vi "controller.vi"(3 "KD":sgl, 6 "Reset":bool, 7 "Parameters":T1={"Stimulus"={"Type"=enum."Off", "Phase"=0.0, "Amplitude"=[0.0, 0.0, 0.0], "Injection point"=enum."Total pose", "Closed loop"=FALSE, "Offset"=[0.0, 0.0, 0.0], "Tip -> world"=TRUE, "Frequency"=0.0, "Length"=0.0}, "Goal Filter A"={"Speedup max"=0.0, "Speedup thresh"=0.15, "Speedup nonlin"=0.0, "Filters"=[]}, "Mode controls"={"Hold"=FALSE, "Cancellation"=FALSE, "Goal filter"=FALSE, "Trigger"=FALSE}, "Manipulator type"=enum."Current piezo", "Manipulator calibration"={"Tool offsets"=[[-0.47364116, -0.25724307, -1.1087934], [0.29673597, -0.25864395, -1.0971603], [-0.04366469, 0.4463568, -1.1035515]], "Tip light calibration"=[[3.2813332, 0.23462732, 0.17832138, -8265.082], [-0.20249099, 2.693321, -0.28150028, -33565.66], [-0.1458117, 0.68216485, 0.8833545, 26862.188], [-1.1202011e-18, 5.861468e-19, 1.7601345e-18, 1.0]], "Handle light calibration"=[], "Base pivots"=[], "Output pivots"=[[0.0, 0.0, -11360.0]], "Length center"=0.0, "Workspace height"=[], "Workspace diameter"=[0.0, 0.0, 36200.0], "Linearization"=[], "Stack travel"=400.0, "Saturation pos"=375.0, "Inverse filters"=[]}, "Network"={"Remote Host"="", "Send Status"=FALSE, "Send Port"=50, "Recv Commands"=FALSE, "Recv Port"=0}, "Goal Filter B"={"Speedup max"=0.0, "Speedup thresh"=0.0, "Speedup nonlin"=0.0, "Filters"=[]}, "Cancellation"={"KP"={"XY"=0.0, "Rxy"=0.0, "Z"=0.0, "Rz"=0.0}, "KI"=2.0, "KD"={"XY"=0.0, "Rxy"=0.0, "Z"=0.0, "Rz"=0.0}, "Max vel"=20.0, "Max acc"=61557.0, "Int error limit"=2.0, "RCM gain"=0.0, "Bypass"=FALSE, "Degraded gain"=0.0}, "Transition time"=0.0, "Estimation"={"Link"={"Measure noise"=[], "Process noise"=[], "Alt process noise"=[], "Alt turnoff cycles"=20, "Innovation limit"=[], "Residue threshold"=0.0, "Enable"=FALSE}, "Handle"={"Measure noise"=[], "Process noise"=[], "State limits"=[], "Innovation limit"=[], "Prediction Lookahead"=0.0, "Enable"=FALSE}}} {"Transition time" format="%_3f"; "Cancellation"."Degraded gain" min=0 max=1 step=0.1 format="%#_3p"; "Cancellation"."RCM gain" min=0 max=1 step=0.1 format="%#_3p"; "Cancellation"."KD"."Rz" min=0 max=1 step=0.1 format="%#_3p"; "Cancellation"."KD"."Rxy" min=0 max=1 step=0.1 format="%#_3p"; "Cancellation"."KD"."Z" min=0 max=1 step=0.1 format="%#_3p"; "Cancellation"."KD"."XY" min=0 max=1 step=0.1 format="%#_3p"; "Cancellation"."KI" min=0 max=1 step=0.01 format="%#_3p"; "Cancellation"."KP"."Rz" min=0 max=1 step=0.1 format="%#_3p"; "Cancellation"."KP"."Rxy" min=0 max=1 step=0.1 format="%#_3p"; "Cancellation"."KP"."Z" min=0 max=1 step=0.1 format="%#_3p"; "Cancellation"."KP"."XY" min=0 max=1 step=0.1 format="%#_3p"; "Cancellation"."Max acc" format="%#_3p"; "Goal Filter B"."Filters"."V limit range" format="%_3p"; "Goal Filter B"."Filters"."V limit" format="%_3p"; "Goal Filter B"."Filters"."Upper Q" format="%_3f"; "Goal Filter B"."Filters"."Upper Fc" format="%_3p"; "Goal Filter B"."Filters"."Lower Q" format="%_3f"; "Goal Filter B"."Filters"."Scale factor" format="%_3f"; "Goal Filter B"."Filters"."Lower Fc" format="%_3p"; "Goal Filter B"."Speedup nonlin" format="%_3p"; "Goal Filter B"."Speedup thresh" format="%_3p"; "Goal Filter B"."Speedup max" format="%_3p"; "Manipulator calibration"."Saturation pos" format="%#.1f"; "Manipulator calibration"."Stack travel" format="%#.1f"; "Manipulator calibration"."Output pivots" format="%#_6f"; "Manipulator calibration"."Base pivots" format="%#_6f"; "Manipulator calibration"."Handle light calibration" format="%#.1f"; "Manipulator calibration"."Tip light calibration" format="%#.1f"; "Goal Filter A"."Filters"."V limit range" format="%_3p"; "Goal Filter A"."Filters"."V limit" format="%_3p"; "Goal Filter A"."Filters"."Upper Q" format="%_3f"; "Goal Filter A"."Filters"."Upper Fc" format="%_3p"; "Goal Filter A"."Filters"."Lower Q" format="%_3f"; "Goal Filter A"."Filters"."Scale factor" format="%_3f"; "Goal Filter A"."Filters"."Lower Fc" format="%_3p"; "Goal Filter A"."Speedup nonlin" format="%_3p"; "Goal Filter A"."Speedup thresh" format="%_3p"; "Goal Filter A"."Speedup max" format="%_3p"; "Stimulus"."Length" min=0.0 max=100.0 step=100.0 format="%#_4p"; "Stimulus"."Frequency" min=0.0 step=100.0 format="%#_4g"; "Stimulus"."Offset" format="%#_3p"; "Stimulus"."Amplitude" format="%#_3p"; "Stimulus"."Phase" min=-180.0 max=360.0 step=100.0 format="%#.2f"}, 8 "Manipulator status":sgl[](array[numeric]), 9 "KI":sgl, 10 "Stack error in":sgl[](array[numeric]), 11 "KP":sgl) -> (4 "Saturation":bool, 5 "Stack commands":sgl[](array[numeric]))   [LabVIEW 2013]
uses:
  testing/Micron params.ctl
  testing/stimulus.ctl
  testing/injection_point.ctl
  filtering/goal_loop_parms.ctl
  testing/mode_conrols.ctl
  testing/manipulator_cal.ctl
  asap/labview/testing/probe_calibration.ctl
  host/network_params.ctl
  sq_control_params.ctl
  decoupled_gain.ctl
  estimation_controls.ctl
panel:
  in  "Last stack error":sgl[](array[numeric])
  in  "Integral error":sgl[](array[numeric])=[0.0, 0.0, 0.0, 0.0, 0.0, 0.0]
  # "Locals:"
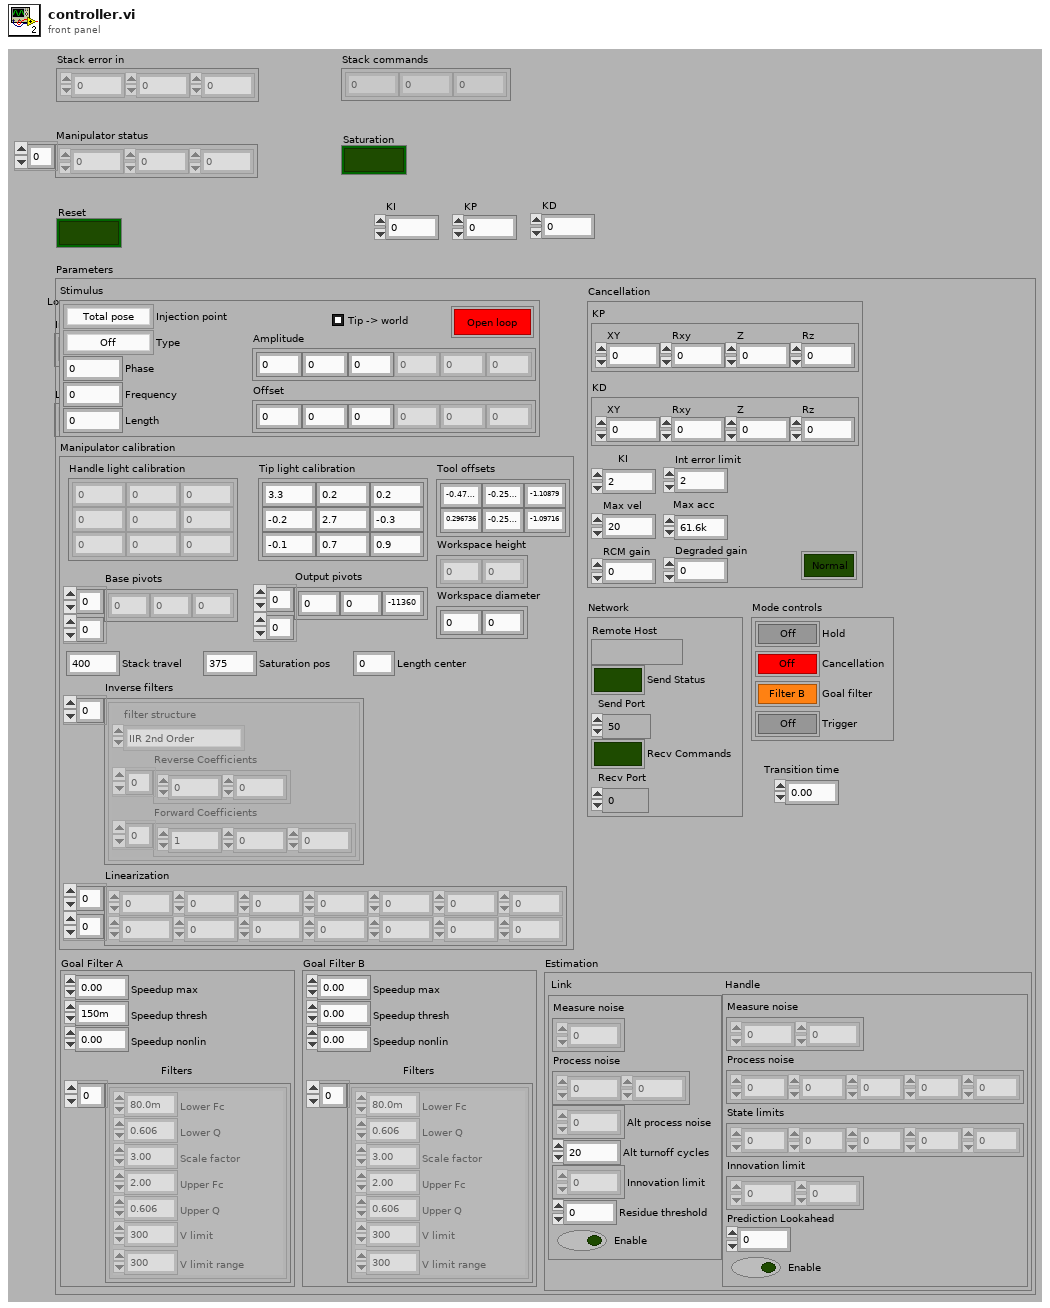
[diagram p1: front panel]
types:
  T1 = typedef "Micron params.ctl" = cluster{"Stimulus":T2, "Goal Filter A":T4, "Mode controls":T5, "Manipulator type":enum16{"Current piezo", "Voltage piezo"}, "Manipulator calibration":T6, "Network":T8, "Goal Filter B":T4, "Cancellation":T9, "Transition time":sgl, "Estimation":T11}
  T2 = typedef "stimulus.ctl" = cluster{"Type":enum16{"Off", "Step", "Sine", "Triangle", "Arbitrary"}, "Phase":dbl, "Amplitude":sgl[], "Injection point":T3, "Closed loop":bool, "Offset":sgl[], "Tip -> world":bool, "Frequency":dbl, "Length":dbl}
  T3 = typedef "injection_point.ctl" = enum16{"Total pose", "V limiter", "Goal ", "Link position", "KF link position", "Inverse kin", "Link goal", "Link error", "Controller", "Output", "Drive", "Light"}
  T4 = typedef "goal_loop_parms.ctl" = cluster{"Speedup max":sgl, "Speedup thresh":sgl, "Speedup nonlin":sgl, "Filters":cluster{"Lower Fc":sgl, "Lower Q":sgl, "Scale factor":sgl, "Upper Fc":sgl, "Upper Q":sgl, "V limit":sgl, "V limit range":sgl}[]}
  T5 = typedef "mode_conrols.ctl" = cluster{"Hold":bool, "Cancellation":bool, "Goal filter":bool, "Trigger":bool}
  T6 = typedef "manipulator_cal.ctl" = cluster{"Tool offsets":sgl[][], "Tip light calibration":T7, "Handle light calibration":T7, "Base pivots":sgl[][], "Output pivots":sgl[][], "Length center":sgl, "Workspace height":sgl[], "Workspace diameter":sgl[], "Linearization":sgl[][], "Stack travel":sgl, "Saturation pos":sgl, "Inverse filters":cluster{"filter structure":enum32{"IIR 2nd Order", "IIR 4th Order"}, "Reverse Coefficients":dbl[], "Forward Coefficients":dbl[]}[]}
  T7 = typedef "probe_calibration.ctl" = sgl[][]
  T8 = typedef "network_params.ctl" = cluster{"Remote Host":string, "Send Status":bool, "Send Port":u16, "Recv Commands":bool, "Recv Port":u16}
  T9 = typedef "sq_control_params.ctl" = cluster{"KP":T10, "KI":sgl, "KD":T10, "Max vel":sgl, "Max acc":sgl, "Int error limit":sgl, "RCM gain":sgl, "Bypass":bool, "Degraded gain":sgl}
  T10 = typedef "decoupled_gain.ctl" = cluster{"XY":sgl, "Rxy":sgl, "Z":sgl, "Rz":sgl}
  T11 = typedef "estimation_controls.ctl" = cluster{"Link":cluster{"Measure noise":dbl[], "Process noise":dbl[], "Alt process noise":dbl[], "Alt turnoff cycles":i32, "Innovation limit":dbl[], "Residue threshold":dbl, "Enable":bool}, "Handle":cluster{"Measure noise":dbl[], "Process noise":dbl[], "State limits":dbl[], "Innovation limit":dbl[], "Prediction Lookahead":sgl, "Enable":bool}}
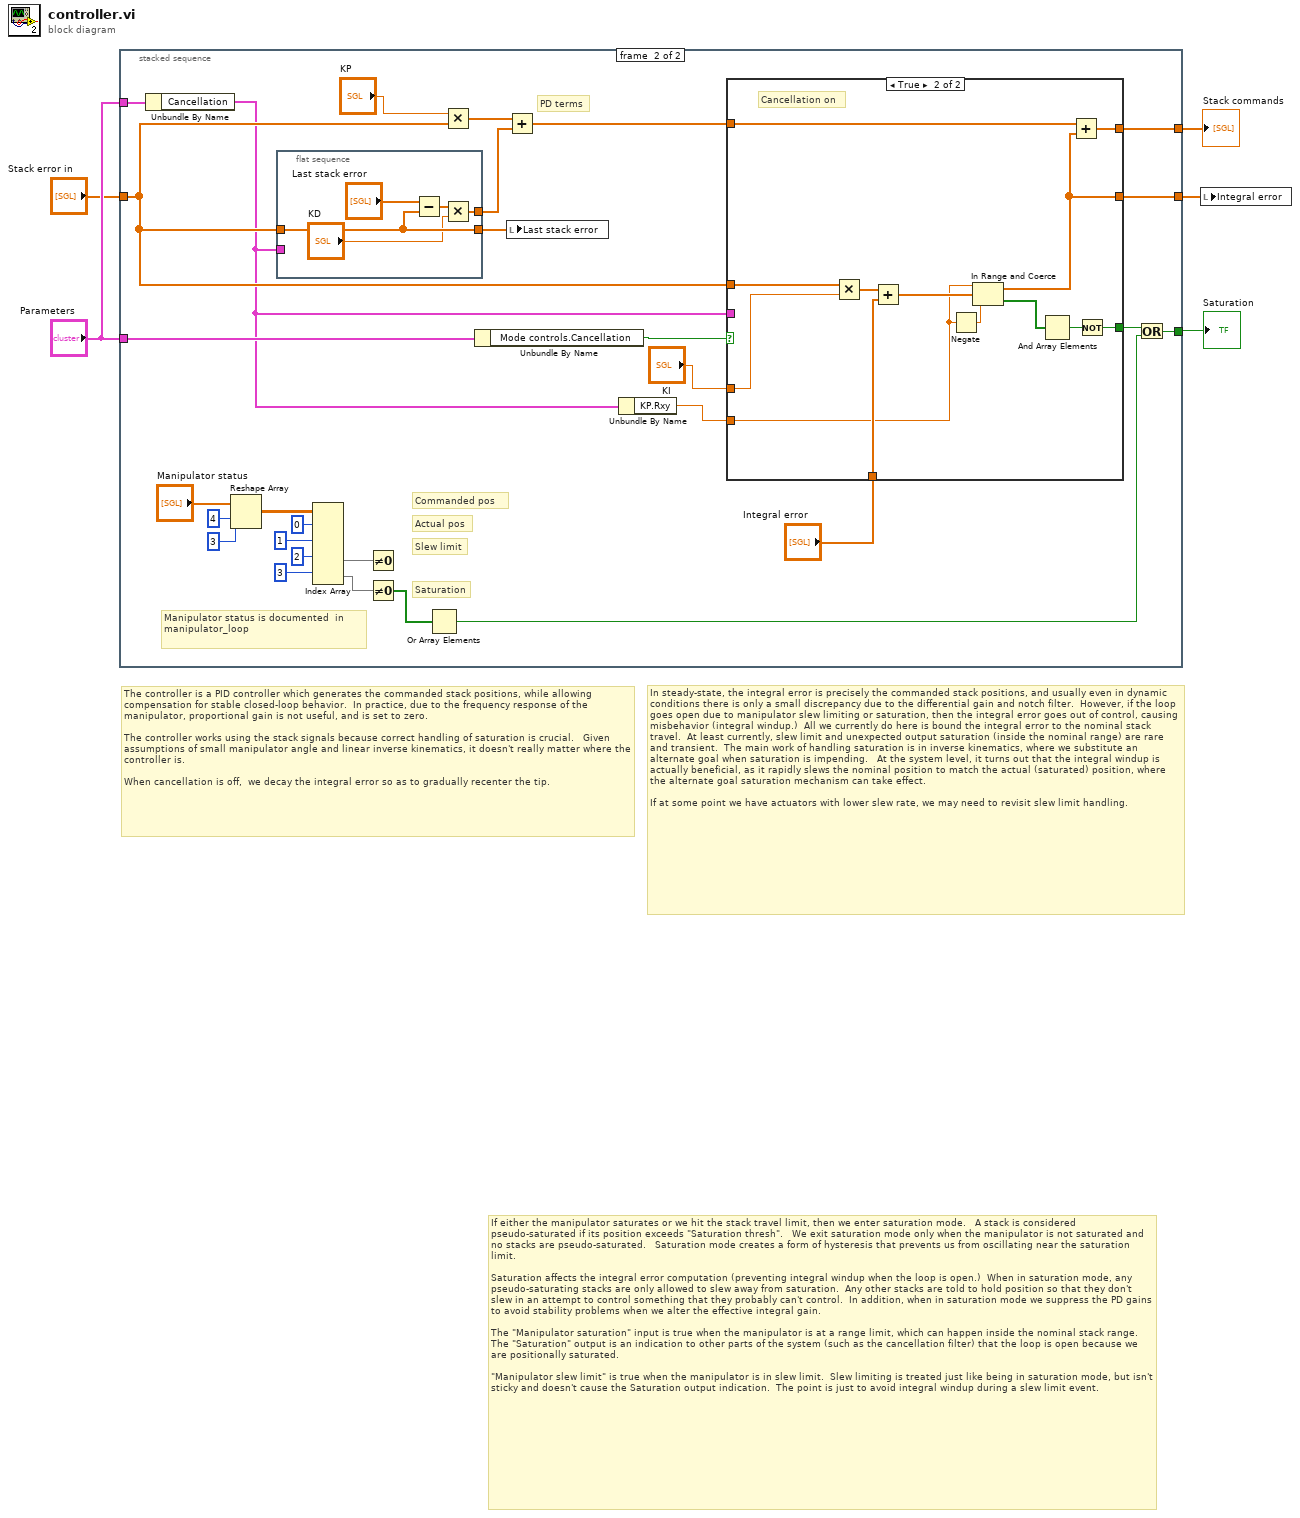
[diagram p0: block diagram]
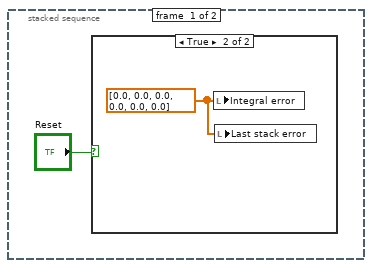
[diagram p2: hidden frame]
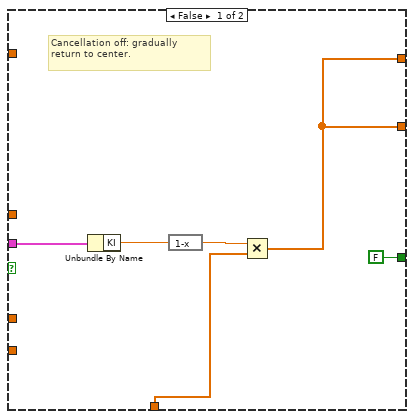
[diagram p4: hidden frame]
diagram:
  # "In steady-state, the integral error is precisely the commanded stack positions, and usually even in dynamic conditions there is only a small discrepancy due to the differential gain and notch filter.  However, if the loop goes open due to manipulator slew limiting or saturation, then the integral error goes out of control, causing  misbehavior (integral windup.)  All we currently do here is bound the integral error to the nominal stack travel.  At least currently, slew limit and unexpected output saturation (inside the nominal range) are rare and transient.  The main work of handling saturation is in inverse kinematics, where we substitute an alternate goal when saturation is impending.   At the system level, it turns out that the integral windup is actually beneficial, as it rapidly slews the nominal position to match the actual (saturated) position, where the alternate goal saturation mechanism can take effect.\n\nIf at some point we have actuators with lower slew rate, we may need to revisit slew limit handling."
  # "If either the manipulator saturates or we hit the stack travel limit, then we enter saturation mode.   A stack is considered pseudo-saturated if its position exceeds \"Saturation thresh\".   We exit saturation mode only when the manipulator is not saturated and no stacks are pseudo-saturated.   Saturation mode creates a form of hysteresis that prevents us from oscillating near the saturation limit.  \n\nSaturation affects the integral error computation (preventing integral windup when the loop is open.)  When in saturation mode, any  pseudo-saturating stacks are only allowed to slew away from saturation.  Any other stacks are told to hold position so that they don't slew in an attempt to control something that they probably can't control.  In addition, when in saturation mode we suppress the PD gains to avoid stability problems when we alter the effective integral gain.\n\nThe \"Manipulator saturation\" input is true when the manipulator is at a range limit, which can happen inside the nominal stack range. The \"Saturation\" output is an indication to other parts of the system (such as the cancellation filter) that the loop is open because we are positionally saturated.  \n\n\"Manipulator slew limit\" is true when the manipulator is in slew limit.  Slew limiting is treated just like being in saturation mode, but isn't sticky and doesn't cause the Saturation output indication.  The point is just to avoid integral windup during a slew limit event."
  # "The controller is a PID controller which generates the commanded stack positions, while allowing compensation for stable closed-loop behavior.  In practice, due to the frequency response of the manipulator, proportional gain is not useful, and is set to zero. \n\nThe controller works using the stack signals because correct handling of saturation is crucial.   Given assumptions of small manipulator angle and linear inverse kinematics, it doesn't really matter where the controller is.\n\nWhen cancellation is off,  we decay the integral error so as to gradually recenter the tip."
  n1 = stacked-sequence {
    tunnel: "Stack error in" -> [_ w31]
    tunnel: "Parameters" -> [_ w33]
    tunnel: [_ w29] -> w3
    tunnel: "Parameters" -> [_ w22]
    tunnel: [_ w21] -> w2
    tunnel: [_ w20] -> w1
    frame #0 {
      n2 = case shown="True" "Reset" {
        frame False {
        }
        frame True {
          w7 = sgl[] [0.0, 0.0, 0.0, 0.0, 0.0, 0.0] ("Integral error")
          n3 = local write "Integral error"(w7) -> ()
          n4 = local write "Last stack error"(w7) -> ()
        }
      }
    }
    frame #1 {
      # "Actual pos"
      # "Commanded pos"
      # "Saturation"
      # "Slew limit"
      # "Manipulator status is documented  in manipulator_loop"
      # "PD terms"
      n5 = Unbundle By Name(w22) -> ("Cancellation"=w11:T9)
      n6 = Reshape Array("Manipulator status", 4 ("dimension size"), 3 ("dimension size")) -> (w26:sgl[][])
      n7 = flat-sequence {
        tunnel: w11 -> [_]
        tunnel: [w59] -> w35
        tunnel: w31 -> [w58]
        tunnel: [w58] -> w34
        frame #0 {
          n8 = Subtract(x="Last stack error", y=w58) -> (x-y=w60:sgl[])
          n9 = Multiply(x=w60, y="KD") -> (x*y=w59:sgl[])
        }
      }
      n10 = Index Array(array=w26, index (row) #1=0 ("index (row)"), index (row) #2=1 ("index (row)"), index (row) #3=2 ("index (row)"), index (row) #4=3 ("index (row)")) -> (element #3=w27:sgl[], element #4=w28:sgl[])  [unwired: 4 in, 2 out]
      n11 = Not Equal To 0?(x=w27) -> ()  [unwired: 1 out]
      n12 = Not Equal To 0?(x=w28) -> (x != 0?=w13:bool[])
      n13 = Or Array Elements(Boolean array=w13) -> (logical OR=w18:bool)
      n14 = Multiply(x="KP", y=w31) -> (x*y=w36:sgl[])
      n15 = Unbundle By Name(w33) -> ("Mode controls.Cancellation"=w32:bool)
      n16 = Add(x=w36, y=w35) -> (x+y=w30:sgl[])
      n17 = local write "Last stack error"(w34) -> ()
      n18 = Unbundle By Name(w11) -> ("KP.Rxy"=w12:sgl)
      n19 = case shown="True" w32 {
        tunnel: [w40 w52] -> w21
        tunnel: w31 -> [_ w53]
        tunnel: w30 -> [_ w44]
        tunnel: [w40 w51] -> w29
        tunnel: "Integral error" -> [w39 w50]
        tunnel: [FALSE w47] -> w19
        tunnel: "KI" -> [_ w46]
        tunnel: w12 -> [_ w45]
        tunnel: w11 -> [w37 _]
        frame False {
          # "Cancellation off: gradually return to center."
          n20 = Unbundle By Name(w37) -> ("KI"=w42:sgl)
          n21 = expression code="1-x"(w42) -> (w41:sgl)
          n22 = Multiply(x=w41, y=w39) -> (x*y=w40:sgl[])
        }
        frame True {
          # "Cancellation on"
          n23 = Multiply(x=w53, y=w46) -> (x*y=w43:sgl[])
          n24 = Add(x=w43, y=w50) -> (x+y=w54:sgl[])
          n25 = Negate(x=w45) -> (-x=w55:sgl)
          n26 = In Range and Coerce(upper limit=w45, x=w54, lower limit=w55) -> (coerced(x)=w52:sgl[], In Range?=w49:bool[])
          n27 = And Array Elements(Boolean array=w49) -> (logical AND=w48:bool)
          n28 = Add(x=w44, y=w52) -> (x+y=w51:sgl[])
          n29 = Not(x=w48) -> (.not. x?=w47:bool)
        }
      }
      n30 = Or(x=w19, y=w18) -> (x .or. y?=w20:bool)
    }
  }
  "Saturation" <- w1
  "Stack commands" <- w3
  n31 = local write "Integral error"(w2) -> ()
